vi "Add Custom NumberingFormat.vi"(8 "error in":errorcluster, 10 "Format":string, 11 "Spreadsheet Doc in":refnum<k24>) -> (0 "error out":errorcluster, 2 "StyleIndex":u32, 3 "SpreadsheetDoc out":refnum<k24>)   [LabVIEW 2021, in "Open Xml.lvlib"]
uses:
  Open Xml.lvlib
  D:/git/Open-Xml-LabVIEW/dll/DocumentFormat.OpenXml.dll
  dll/DocumentFormat.OpenXml.dll
  D:/git/Open-Xml-LabVIEW/dll/DocumentFormat.OpenXml.Framework.dll
  dll/DocumentFormat.OpenXml.Framework.dll
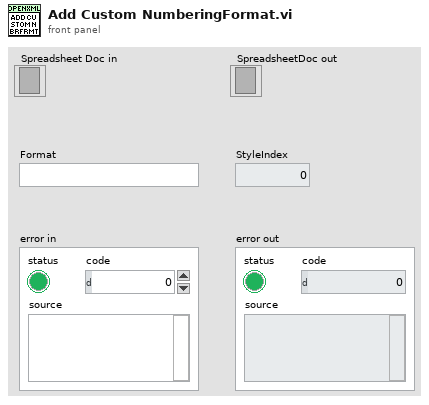
[diagram p1: front panel]
types:
  T1 = cluster{"NumberFormatId":u32, "FontId":u32, "FillId":u32, "BorderId":u32, "FormatId":u32, "ApplyNumberFormat":bool}
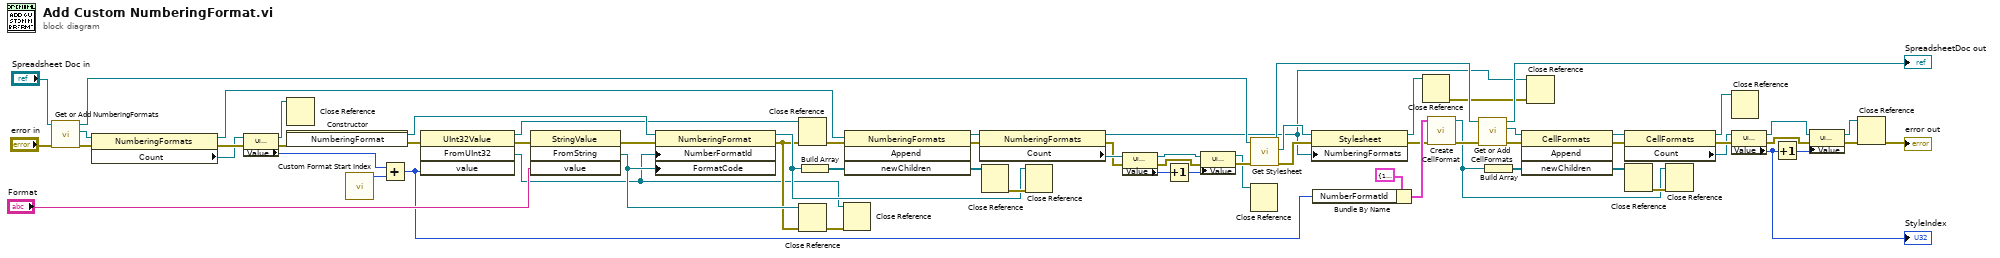
[diagram p0: block diagram]
diagram:
  n1 = call "Get or Add NumberingFormats.vi"("error in"="error in", "SpreadsheetDoc in"="Spreadsheet Doc in") -> ("error out"=w16:errorcluster, "NumberingFormats"=w12:refnum<k24>, "SpreadsheetDoc out"=w14:refnum<k24>)  [unwired: 7 in]
  n2 = property class="NumberingFormats"(reference=w12, error in=w16) -> (reference out=w11:refnum<k24>, error out=w13:errorcluster, "Count"=w10:refnum<k24>)
  n3 = property class="UInt32Value"(reference=w10, error in=w13) -> (reference out=w7:refnum<k24>, error out=w8:errorcluster, "Value"=w9:u32)
  n4 = Close Reference(reference=w7) -> ()  [unwired: 1 in, 1 out]
  n5 = constructor class="NumberingFormat"(error in=w8) -> (reference out=w58:refnum<k24>, error out=w60:errorcluster)  [unwired: 2 in, 1 out]
  n6 = call "Custom Format Start Index.vi"() -> ("Start ID"=w59:u32)  [unwired: 11 in]
  n7 = Add(x=w9, y=w59) -> (x+y=w25:u32)
  n8 = invoke class="UInt32Value" method="FromUInt32"(error in=w60, "value"=w25) -> (reference out=w39:refnum<k24>, error out=w61:errorcluster, "FromUInt32"=w1:refnum<k24>)  [unwired: 2 in, 1 out]
  n9 = invoke class="StringValue" method="FromString"(error in=w61, "value"="Format") -> (error out=w62:errorcluster, "FromString"=w4:refnum<k24>)  [unwired: 2 in, 2 out]
  n10 = property class="NumberingFormat"(reference=w58, error in=w62, "NumberFormatId"=w1, "FormatCode"=w4) -> (reference out=w17:refnum<k24>, error out=w3:errorcluster)
  n11 = Close Reference(reference=w39, error in (no error)=w3) -> (error out=w40:errorcluster)
  n12 = Close Reference(reference=w4, error in (no error)=w3) -> (error out=w2:errorcluster)
  n13 = Build Array(w17) -> (w22:refnum<k24>[])
  n14 = Close Reference(reference=w1, error in (no error)=w2) -> ()  [unwired: 1 out]
  n15 = invoke class="NumberingFormats" method="Append"(reference=w11, error in=w40, "newChildren"=w22) -> (reference out=w56:refnum<k24>, error out=w57:errorcluster, "newChildren"=w24:refnum<k24>[])  [unwired: 1 in, 1 out]
  n16 = property class="NumberingFormats"(reference=w56, error in=w57) -> (reference out=w5:refnum<k24>, error out=w54:errorcluster, "Count"=w55:refnum<k24>)
  n17 = Close Reference(reference=w24) -> (error out=w23:errorcluster)  [unwired: 1 in]
  n18 = Close Reference(reference=w17, error in (no error)=w23) -> ()  [unwired: 1 out]
  n19 = property class="UInt32Value"(reference=w55, error in=w54) -> (reference out=w50:refnum<k24>, error out=w51:errorcluster, "Value"=w53:u32)
  n20 = Increment(x=w53) -> (x+1=w52:u32)
  n21 = property class="UInt32Value"(reference=w50, error in=w51, "Value"=w52) -> (reference out=w47:refnum<k24>, error out=w48:errorcluster)
  n22 = Close Reference(reference=w47) -> ()  [unwired: 1 in, 1 out]
  n23 = call "Get Stylesheet.vi"("error in"=w48, "SpreadsheetDoc in"=w14) -> ("error out"=w46:errorcluster, "Stylesheet"=w49:refnum<k24>, "SpreadsheetDoc out"=w44:refnum<k24>)  [unwired: 7 in]
  n24 = property class="Stylesheet"(reference=w49, error in=w46, "NumberingFormats"=w5) -> (reference out=w41:refnum<k24>, error out=w27:errorcluster)
  n25 = Bundle By Name(cluster=T1 {"NumberFormatId"=164, "FontId"=0, "FillId"=0, "BorderId"=0, "FormatId"=0, "ApplyNumberFormat"=TRUE} ("Format"), "NumberFormatId"=w25) -> (w28:T1)
  n26 = Close Reference(reference=w41) -> (error out=w6:errorcluster)  [unwired: 1 in]
  n27 = call "Create CellFormat.vi"("error in"=w27, "Formats"=w28) -> ("error out"=w26:errorcluster, "CellFormat"=w18:refnum<k24>)  [unwired: 8 in]
  n28 = call "Get or Add CellFormats.vi"("error in"=w26, "SpreadsheetDoc in"=w44) -> ("error out"=w45:errorcluster, "CellFormats"=w42:refnum<k24>, "SpreadsheetDoc out"=→"SpreadsheetDoc out":refnum<k24>)  [unwired: 7 in]
  n29 = Build Array(w18) -> (w19:refnum<k24>[])
  n30 = invoke class="CellFormats" method="Append"(reference=w42, error in=w45, "newChildren"=w19) -> (reference out=w38:refnum<k24>, error out=w43:errorcluster, "newChildren"=w21:refnum<k24>[])  [unwired: 1 in, 1 out]
  n31 = Close Reference(reference=w5, error in (no error)=w6) -> ()  [unwired: 1 out]
  n32 = property class="CellFormats"(reference=w38, error in=w43) -> (reference out=w31:refnum<k24>, error out=w34:errorcluster, "Count"=w33:refnum<k24>)
  n33 = Close Reference(reference=w21) -> (error out=w20:errorcluster)  [unwired: 1 in]
  n34 = Close Reference(reference=w18, error in (no error)=w20) -> ()  [unwired: 1 out]
  n35 = Close Reference(reference=w31) -> ()  [unwired: 1 in, 1 out]
  n36 = property class="UInt32Value"(reference=w33, error in=w34) -> (reference out=w35:refnum<k24>, error out=w36:errorcluster, "Value"=w65:u32)
  "StyleIndex" <- w65
  n37 = Increment(x=w65) -> (x+1=w37:u32)
  n38 = property class="UInt32Value"(reference=w35, error in=w36, "Value"=w37) -> (reference out=w32:refnum<k24>, error out=w30:errorcluster)
  n39 = Close Reference(reference=w32, error in (no error)=w30) -> (error out=→"error out":errorcluster)
